vi "Fetch Measurement Data.vi"(8 "error in (no error)":errorcluster, 11 "VISA resource name":refnum<visa-resource-name>) -> (0 "error out":errorcluster, 1 "Secondary Parameter":dbl, 2 "Primary Parameter":dbl, 3 "VISA resource name out":refnum<visa-resource-name>, 5 "Data Status":i32)   [LabVIEW 2019, in "Agilent E4980.lvlib"]
doc: "Returns the measurement results with the selected measurement function."
uses:
  Agilent E4980.lvlib
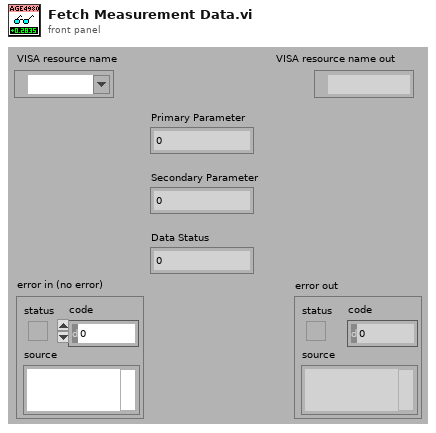
[diagram p1: front panel]
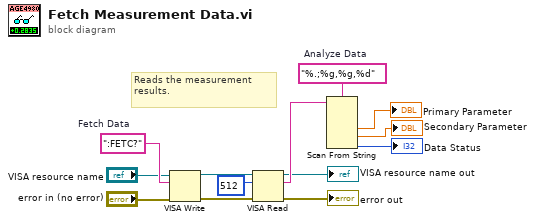
[diagram p0: block diagram]
diagram:
  w6 = "%.;%g,%g,%d"  # Analyze Data
  w13 = ":FETC?"  # Fetch Data
  # "Reads the measurement\nresults."
  n1 = VISA Write(VISA resource name="VISA resource name", write buffer=w13, error in (no error)="error in (no error)") -> (VISA resource name out=w10:refnum<visa-resource-name>, error out=w9:errorcluster)  [unwired: 1 out]
  n2 = VISA Read(VISA resource name=w10, byte count=u32 512, error in (no error)=w9) -> (VISA resource name out=→"VISA resource name out":refnum<visa-resource-name>, read buffer=w7:string, error out=→"error out":errorcluster)  [unwired: 1 out]
  n3 = Scan From String(format string=w6, input string=w7) -> (output 1=→"Primary Parameter":dbl, output 2=→"Secondary Parameter":dbl, output 3=→"Data Status":i32)  [unwired: 5 in, 3 out]
